vi "Connect to Slave.vi"(8 "error in (no error)":errorcluster, 11 "SMSD in":refnum<class "SMSD.lvclass">) -> (0 "error out":errorcluster, 3 "SMSD out":refnum<class "SMSD.lvclass">)   [LabVIEW 2021, in "SMSD.lvclass"]
uses:
  SMSD.lvclass
  D:/my_projects/projects/Algorithms/Labview/21/Master CR/Master CR.lvclass
  Master CR.lvclass/Master CR.ctl
  SMSD.lvclass/SMSD.ctl
  Data Unit/SMSD Data Unit/SMSD Data Unit.lvclass/SMSD Data Unit.ctl
  Network Protocol/SMSD Master/SMSD Master.lvclass/SMSD Master.ctl
  Transmission Data Unit/SMSD/SMSD ADU.lvclass/SMSD ADU.ctl
  Data Unit/SMSD Data Unit/Construct PDU.vi
  Network Protocol/SMSD Master/Read write Master.vi
  Data Unit/SMSD Data Unit/Deconstruct PDU.vi
  Network Protocol/Read Network Protocol.vi
  Transmission Data Unit/SMSD/Write ADU Packet.vi
  Transmission Data Unit/SMSD/Read ADU Packet.vi
  Modbus_v121c/Network Interface/TCP Interface/TCP Shared Components/TCP Write.vi
  Data Unit/SMSD Data Unit/Flatten PDU.vi
  Data Unit/SMSD Data Unit/Unflatten to PDU.vi
  Modbus_v121c/Network Interface/TCP Interface/TCP Shared Components/TCP Read.vi
  <vilib>/Utility/error.llb/Clear Errors.vi
  Network Protocol/SMSD Master/SMSD Master.lvclass
  D:/my_projects/projects/Algorithms/Labview/21/Modbus_v121c/Network Protocol/Network Protocol.lvclass
  Data Unit/SMSD Data Unit/SMSD Data Unit.lvclass
  Master CR.lvclass
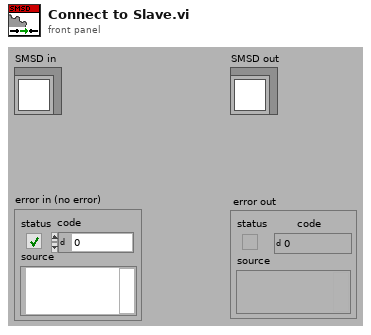
[diagram p1: front panel]
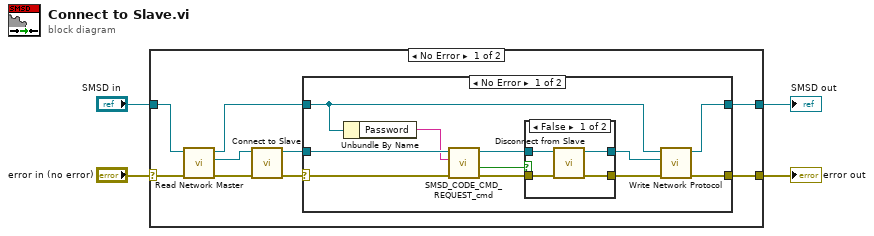
[diagram p0: block diagram]
diagram:
  n1 = case shown="No Error" "error in (no error)" {
    selector: "error in (no error)" -> [w9 w34]
    tunnel: "SMSD in" -> [w11 w33]
    tunnel: [w13 w34] -> w4
    tunnel: [w12 w33] -> w1
    frame No Error {
      n2 = call "Read Network Master.vi"("error in (no error)"=w9, "SMSD in"=w11) -> ("error out"=w8:errorcluster, "TCP Master"=w7:refnum<class "SMSD Master.lvclass">, "SMSD out"=w10:refnum<class "SMSD.lvclass">)  [unwired: 7 in]
      n3 = call-dynamic "Connect to Slave.vi"("error in (no error)"=w8, "TCP master in"=w7) -> ("error out"=w6:errorcluster, "TCP master out"=w5:refnum<class "SMSD Master.lvclass">)  [unwired: 8 in]
      n4 = case shown="No Error" w6 {
        selector: w6 -> [w24 w31]
        tunnel: [w14 w31] -> w13
        tunnel: [w15 w32] -> w12
        tunnel: w10 -> [w16 w32]
        tunnel: w5 -> [w23 _]
        frame No Error {
          n5 = Unbundle By Name(w16) -> ("Password"=w22:string)
          n6 = call "SMSD_CODE_CMD_REQUEST_cmd.vi"("error in (no error)"=w24, "Password"=w22, "SMSD in"=w23) -> ("error out"=w20:errorcluster, "PDU valid?"=w19:bool, "SMSD out"=w21:refnum<class "SMSD Master.lvclass">)  [unwired: 6 in]
          n7 = case shown="False" w19 {
            tunnel: w21 -> [w28 w29]
            tunnel: w20 -> [w27 w30]
            tunnel: [w25 w30] -> w18
            tunnel: [w26 w29] -> w17
            frame False {
              n8 = call-dynamic "Disconnect from Slave.vi"("error in"=w27, "TCP master in"=w28) -> ("error out"=w25:errorcluster, "TCP master out"=w26:refnum<class "SMSD Master.lvclass">)  [unwired: 8 in]
            }
            frame True {
            }
          }
          n9 = call "Write Network Protocol.vi"("error in (no error)"=w18, "Network Protocol"=w17, "Master CR in"=w16) -> ("error out"=w14:errorcluster, "Master CR out"=w15:refnum<class "SMSD.lvclass">)  [unwired: 7 in]
        }
        frame Error {
        }
      }
    }
    frame Error {
    }
  }
  "error out" <- w4
  "SMSD out" <- w1
